vi "Working Window.vi"(8 "error in (no error)":errorcluster, 10 "file path":path=path "D:/Projects/Personal/Multi-LabVIEW-Selector/Multi-LabVIEW Selector.lvproj" caption="打开文件路径", 11 "DB Ref":refnum<class "SharedData.lvclass">) -> (0 "error out":errorcluster, 3 "DB Ref (dup)":refnum<class "SharedData.lvclass">)   [LabVIEW 2014]
uses:
  control/DEF-LabVIEW INFO.ctl
  <vilib>/NEVSTOP/Shared Data Library/SharedData/SharedData.lvclass
  control/DEF-State.ctl
  <vilib>/NEVSTOP/Shared Data Library/SharedData/SharedData.lvclass/SharedData.ctl
  <vilib>/NEVSTOP/Shared Data Library/SharedData/Data operation/_int32.vi
  <vilib>/NEVSTOP/Shared Data Library/SharedData/Data operation/_variant.vi
  <vilib>/NEVSTOP/Shared Data Library/SharedData/support/_[error50002]Invalid DataType.vi
  <vilib>/NEVSTOP/Shared Data Library/SharedData/support/_[error50001]Can't Found Value.vi
  <vilib>/NEVSTOP/Shared Data Library/SharedData/support/_[error50000]Invalid DB REF.vi
  <vilib>/Utility/error.llb/Trim Whitespace.vi
panel:
  out "Symbol Found?":bool
  out "Selected Version":string
  out "Version List":string[](array[string])
  out "Symbol Path":path
  out "Symbol Version":string
  out "LabVIEW Info":T1[](array[typedef])
  in  "Cancel":bool
  in  "OK":bool
  in  "LabVIEW List":string(combo)
  out "CMD line":string caption="命令行参数"
  # "主界面，所有的界面操作都产生消息，推送给Message Framework 处理。"
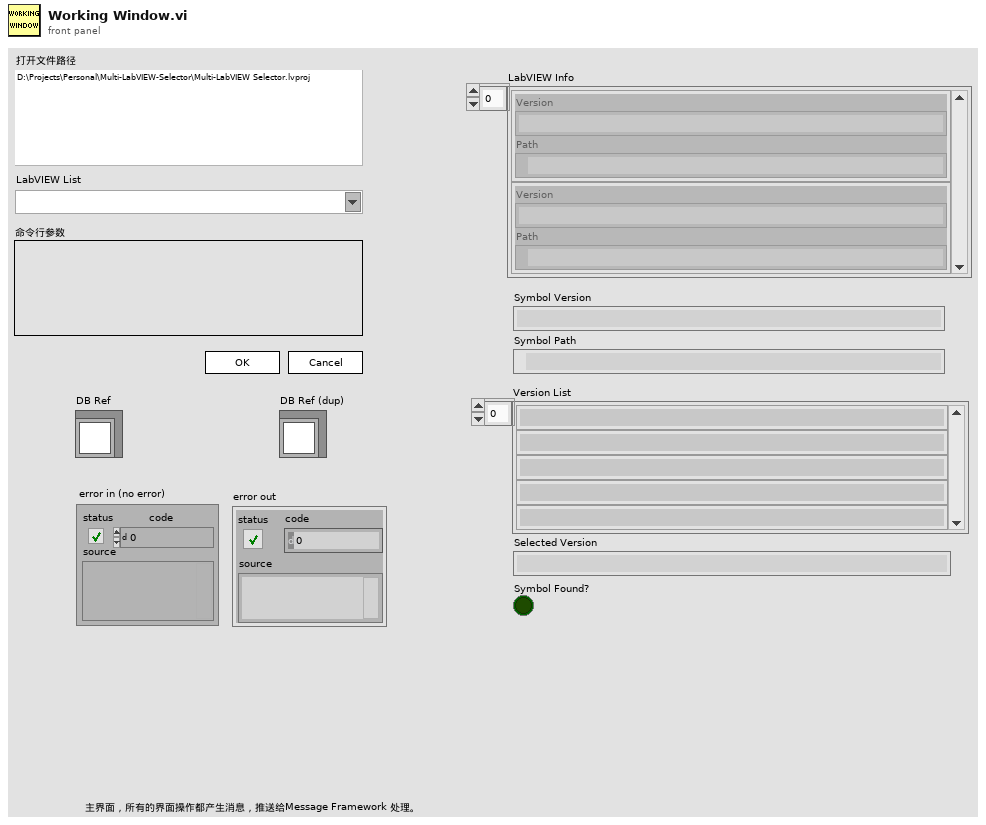
[diagram p1: front panel]
types:
  T1 = typedef "DEF-LabVIEW INFO.ctl" = cluster{"Version":string, "Path":path}
  T2 = typedef "DEF-State.ctl" = enum16{"Get Project Path", "Get Installed LabVIEW Version", "Find New Symbol", "Find Old Symbol", "Replace with New Symbol", "Check If The Symbol Version Exist", "Waiting for User Selection", "Display Information", "Get CMD", "Display CMD", "Excute CMD", "Exit"}
  T3 = cluster{"DB Ref":refnum<class "SharedData.lvclass">, "Project Path":path, "LabVIEW Info":T1[], "Symbol Version":string, "Symbol Path":path, "Version List":string[], "Selected Version":string, "Symbol Found?":bool, "CMD line":string}
  T4 = enum8{"Enabled", "Disabled", "Disabled and Grayed Out"}
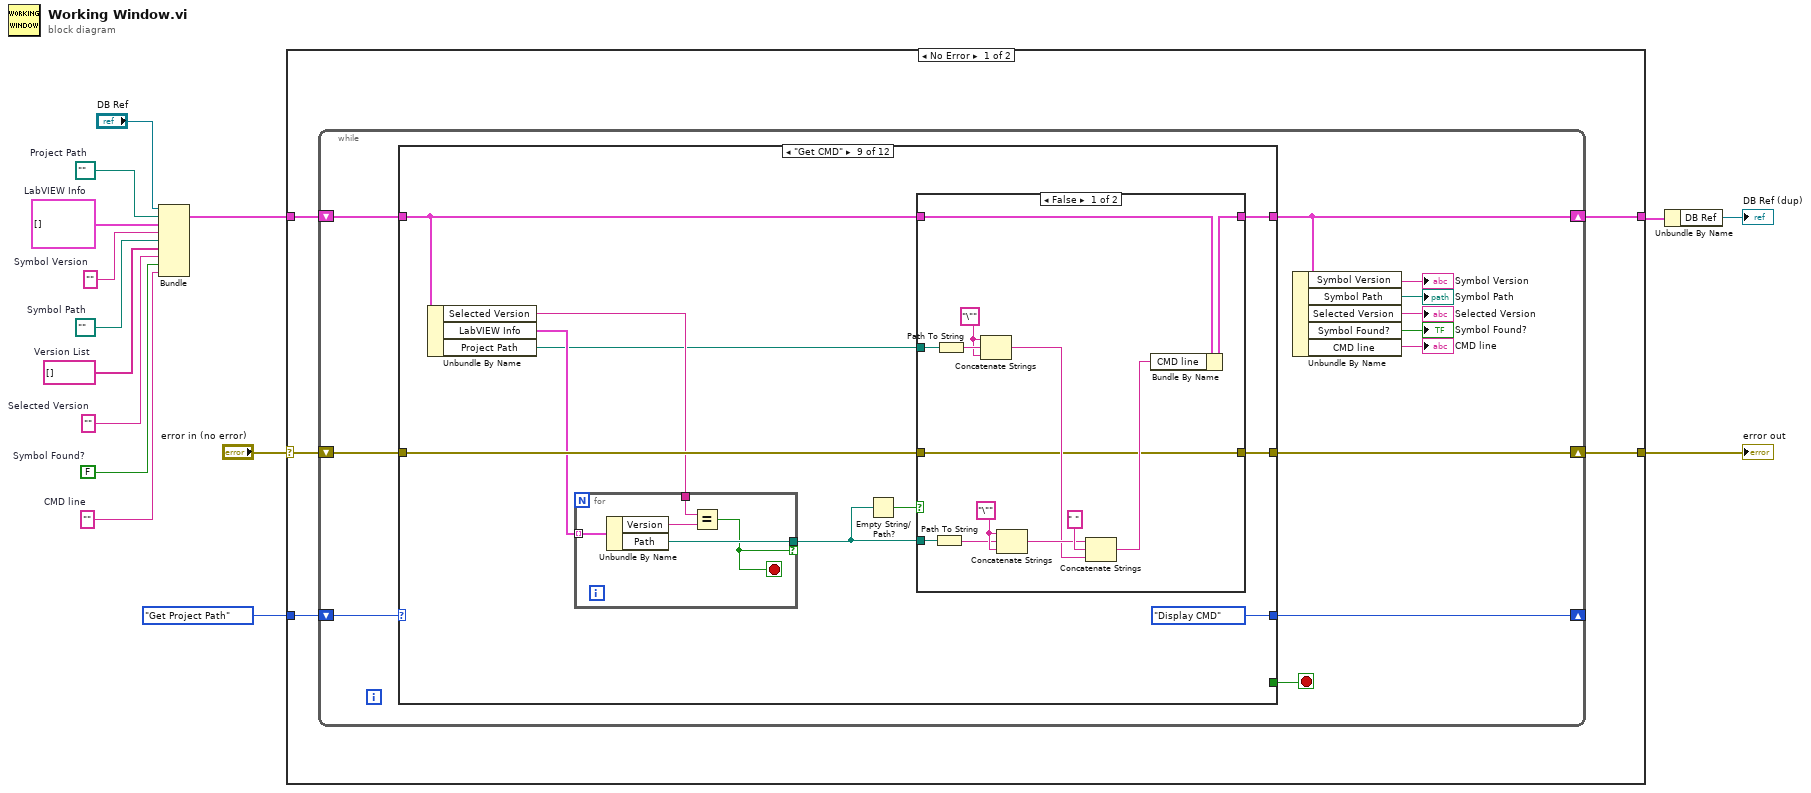
[diagram p0: block diagram]
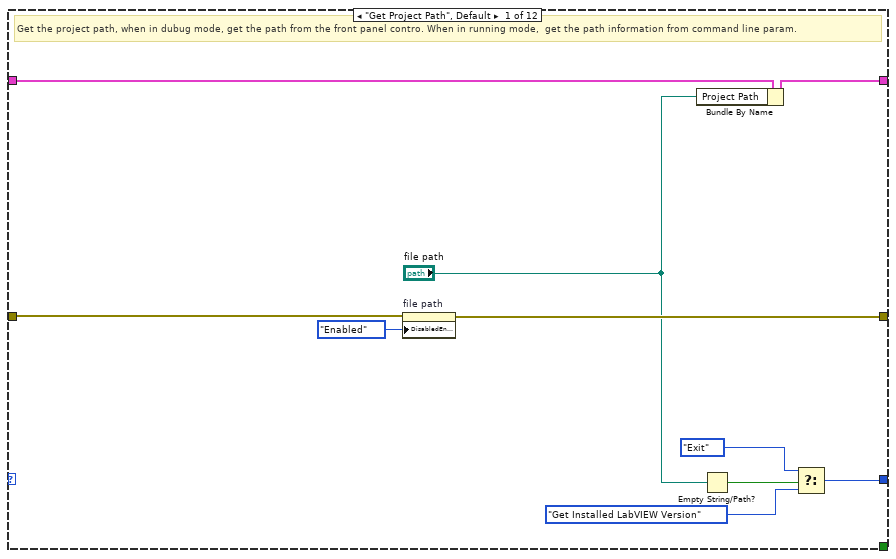
[diagram p2: hidden frame]
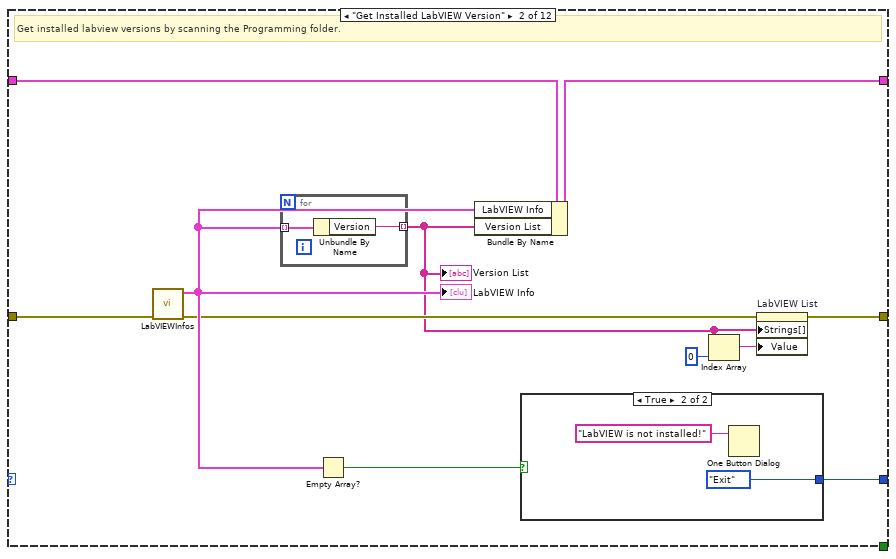
[diagram p3: hidden frame]
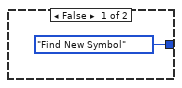
[diagram p4: hidden frame]
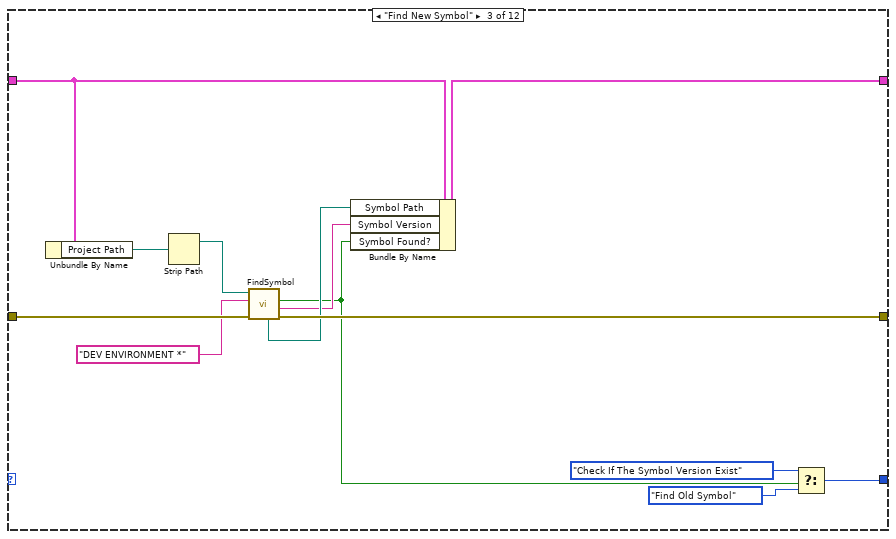
[diagram p5: hidden frame]
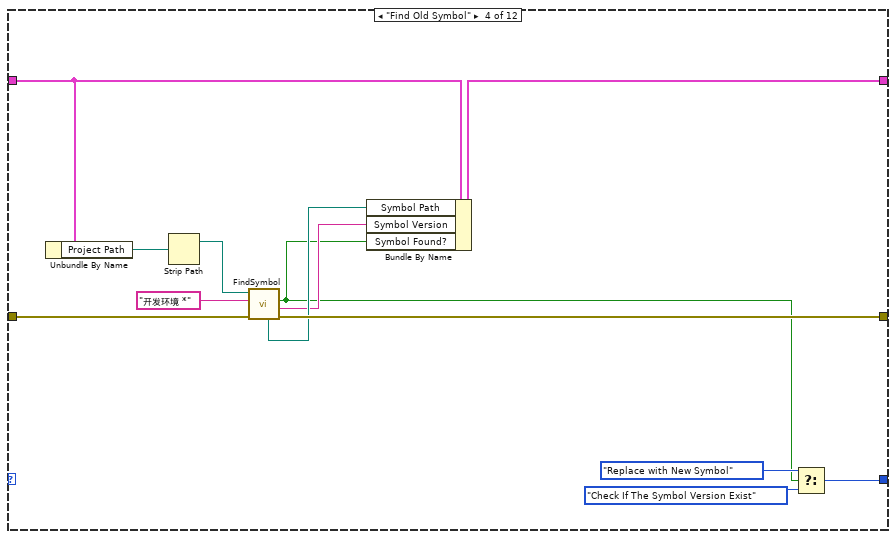
[diagram p6: hidden frame]
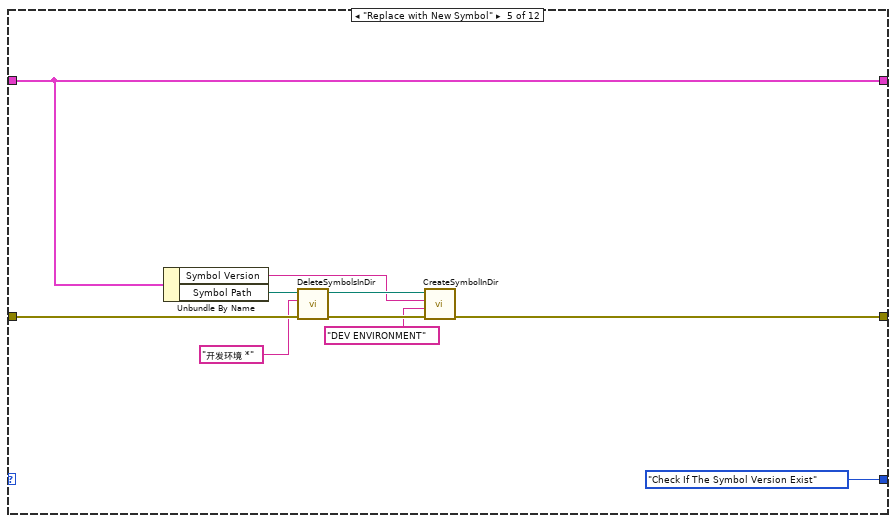
[diagram p7: hidden frame]
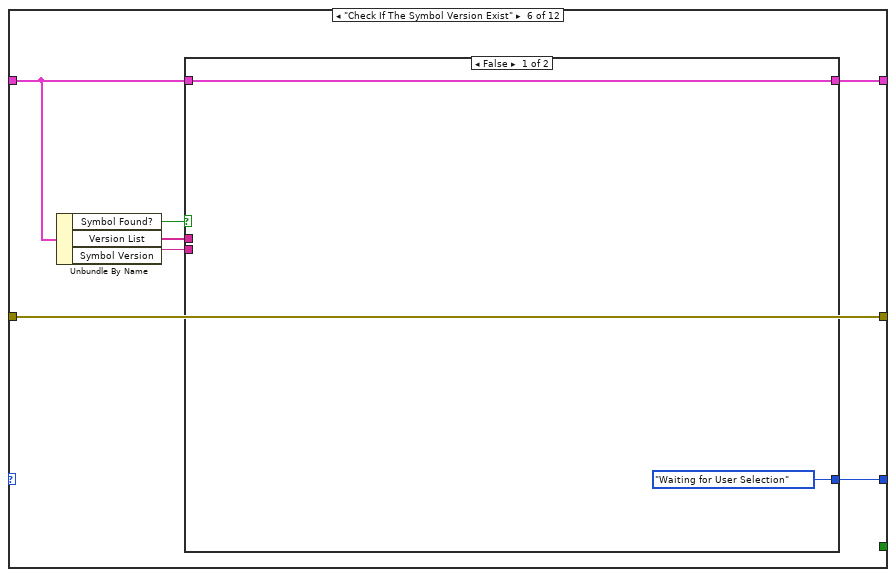
[diagram p8: hidden frame]
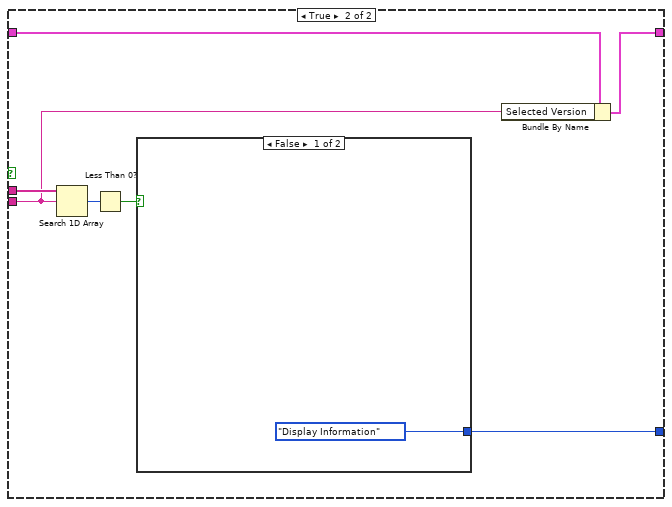
[diagram p9: hidden frame]
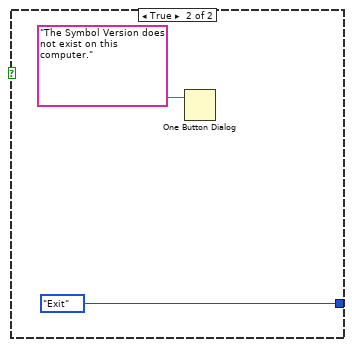
[diagram p10: hidden frame]
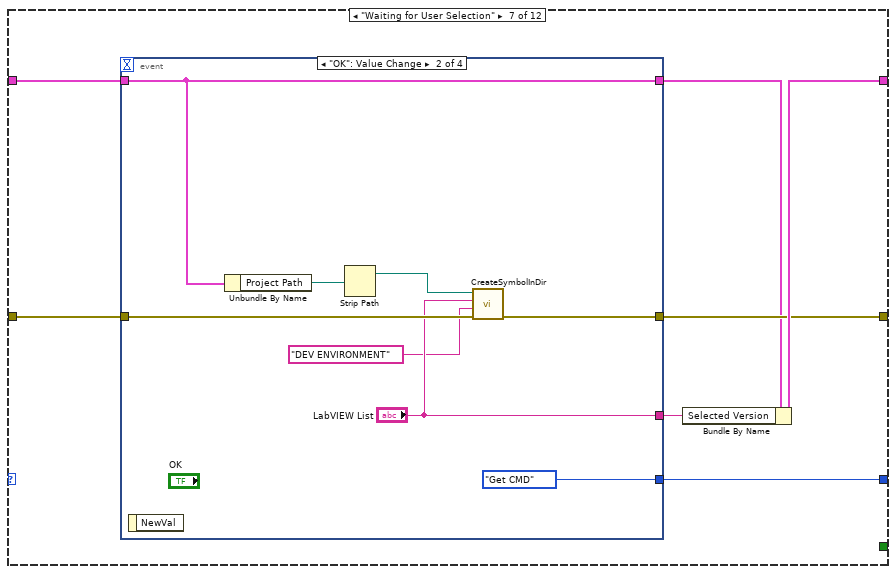
[diagram p11: hidden frame]
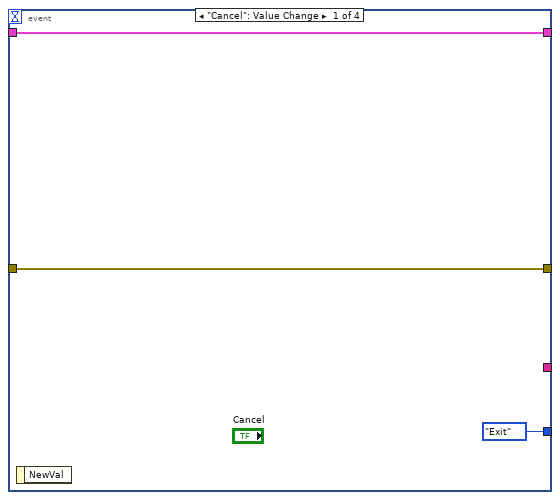
[diagram p12: hidden frame]
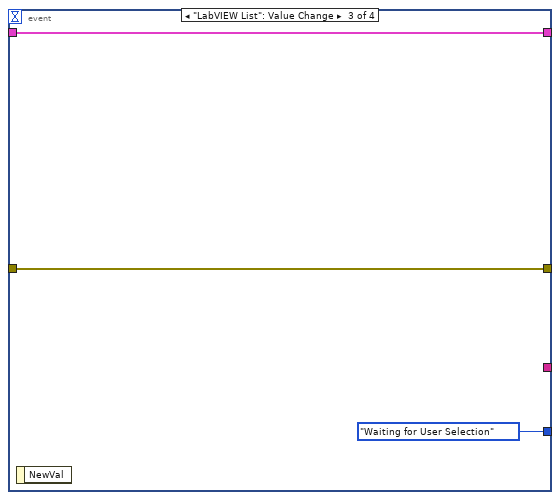
[diagram p13: hidden frame]
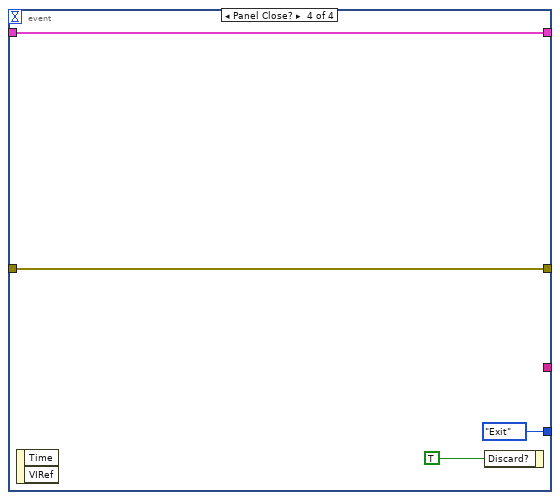
[diagram p14: hidden frame]
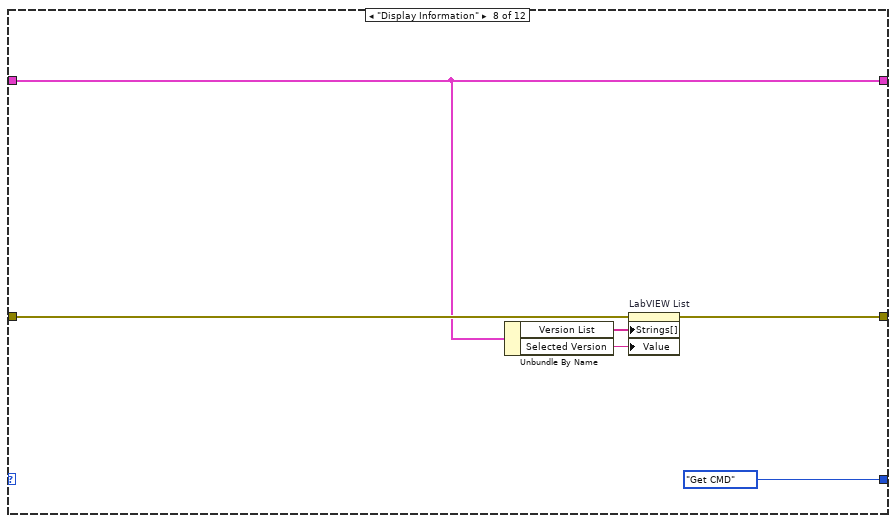
[diagram p15: hidden frame]
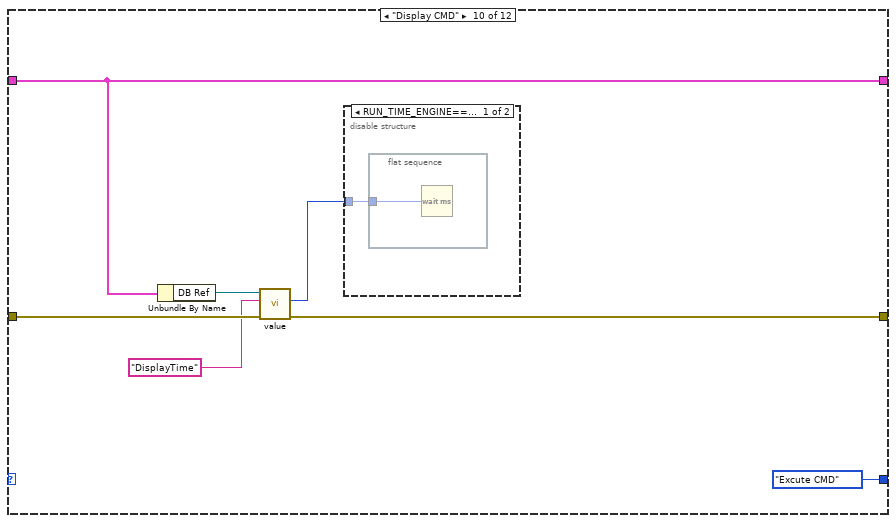
[diagram p17: hidden frame]
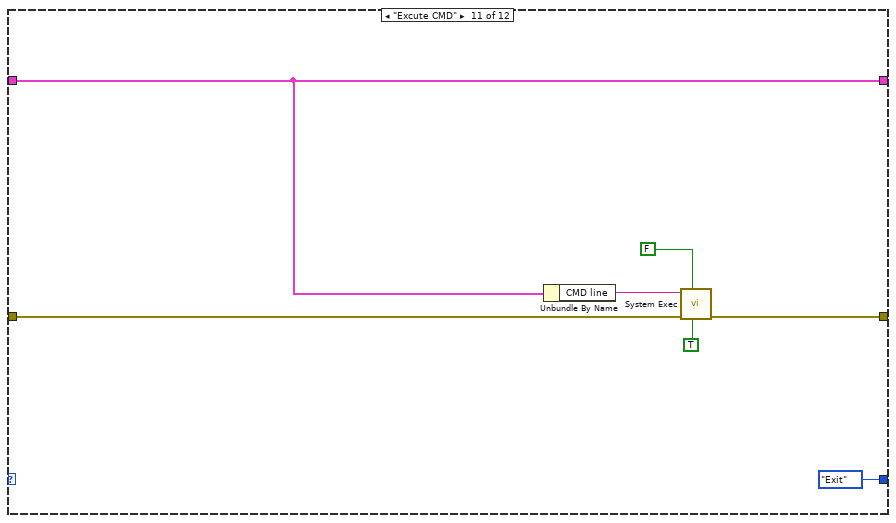
[diagram p19: hidden frame]
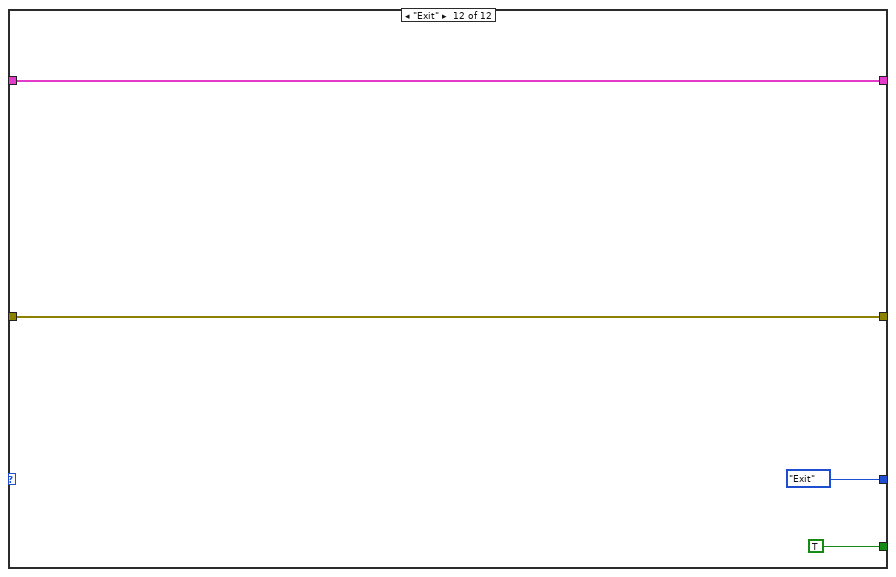
[diagram p20: hidden frame]
diagram:
  w7 = ""  # CMD line
  w8 = FALSE  # Symbol Found?
  w9 = ""  # Selected Version
  w10 = string[] []  # Version List
  w11 = path ""  # Symbol Path
  w12 = ""  # Symbol Version
  w13 = path ""  # Project Path
  w15 = T1[] []  # LabVIEW Info
  n1 = Bundle("DB Ref"="DB Ref", "Project Path"=w13, "LabVIEW Info"=w15, "Symbol Version"=w12, "Symbol Path"=w11, "Version List"=w10, "Selected Version"=w9, "Symbol Found?"=w8, "CMD line"=w7) -> (w14:T3)  [unwired: 1 in]
  n2 = case shown="No Error" "error in (no error)" {
    selector: "error in (no error)" -> [w19 w196]
    tunnel: w14 -> [w20 w195]
    tunnel: [w18 w196] -> w4
    tunnel: [w17 w195] -> w3
    tunnel: DEF-State."Get Project Path" -> [w16 _]
    frame No Error {
      n3 = while {
        shift-right: [w29] -> w18
        shift-left: w19 -> [w30]
        shift-right: [w28] -> _
        shift-left: w16 -> [w32]
        shift-right: [w26] -> w17
        shift-left: w20 -> [w27]
        stop <- w31 stop-if-true
        n4 = case shown="\"Get CMD\"" w32 {
          tunnel: [_ _ _ _ _ _ _ _ _ _ _ TRUE] -> w31
          tunnel: w30 -> [w41 w53 w69 w82 w94 w99 w117 w143 w154 w179 w187 w191]
          tunnel: [w42 w44 w65 w77 w89 w99 w116 w144 w153 w176 w188 w191] -> w29
          tunnel: [w39 w49 w66 w78 DEF-State."Check If The Symbol Version Exist" w98 w118 DEF-State."Get CMD" DEF-State."Display CMD" DEF-State."Excute CMD" DEF-State."Exit" DEF-State."Exit"] -> w28
          tunnel: w27 -> [w36 w52 w64 w76 w93 w96 w115 w142 w146 w180 w185 w192]
          tunnel: [w35 w51 w62 w74 w93 w95 w120 w142 w145 w180 w185 w192] -> w26
          frame "Get Project Path", Default {
            # "Get the project path, when in dubug mode, get the path from the front panel contro. When in running mode,  get the path information from command line param."
            n5 = property on="file path" class="Path"(error in=w41, "DisabledEnum"=T4."Enabled" ("Disabled")) -> (error out=w42:errorcluster)  [unwired: 1 in, 1 out]
            n6 = Bundle By Name(cluster=w36, "Project Path"="file path") -> (w35:T3)
            n7 = Empty String/Path?(string/path="file path") -> (empty?=w40:bool)
            n8 = Select(t=DEF-State."Exit", s=w40, f=DEF-State."Get Installed LabVIEW Version") -> (s? t:f=w39:T2)
          }
          frame "Get Installed LabVIEW Version" {
            # "Get installed labview versions by scanning the Programming folder."
            n9 = call "LabVIEWInfos.vi"("error in (no error)"=w53) -> ("error out"=w45:errorcluster, "LabVIEW Info"=w48:T1[])  [unwired: 9 in]
            "LabVIEW Info" <- w48
            n10 = for {
              tunnel: w48 -> [w55] mode=indexing
              tunnel: [w54] -> w43 mode=indexing
              n11 = Unbundle By Name(w55) -> ("Version"=w54:string)
            }
            "Version List" <- w43
            n12 = Empty Array?(array=w48) -> (empty?=w50:bool)
            n13 = Bundle By Name(cluster=w52, "LabVIEW Info"=w48, "Version List"=w43) -> (w51:T3)
            n14 = case shown="True" w50 {
              tunnel: [DEF-State."Find New Symbol" DEF-State."Exit"] -> w49
              frame False {
              }
              frame True {
                n15 = One Button Dialog(message="LabVIEW is not installed!") -> ()  [unwired: 1 in, 1 out]
              }
            }
            n16 = Index Array(array=w43, index=0) -> (element=w46:string)
            n17 = property on="LabVIEW List" class="CmbBox"(error in=w45, "Strings[]"=w43, "Value"=w46) -> (error out=w44:errorcluster)  [unwired: 1 in, 1 out]
          }
          frame "Find New Symbol" {
            n18 = Unbundle By Name(w64) -> ("Project Path"=w71:path)
            n19 = Strip Path(path=w71) -> (stripped path=w70:path)  [unwired: 1 out]
            n20 = call "FindSymbol.vi"("error in (no error)"=w69, "pattern"="DEV ENVIRONMENT *" ("prefix"), "path"=w70) -> ("error out"=w65:errorcluster, "Version"=w61:string, "Exits?"=w59:bool, "found path"=w63:path)  [unwired: 4 in, 1 out]
            n21 = Bundle By Name(cluster=w64, "Symbol Path"=w63, "Symbol Version"=w61, "Symbol Found?"=w59) -> (w62:T3)
            n22 = Select(t=DEF-State."Check If The Symbol Version Exist", s=w59, f=DEF-State."Find Old Symbol") -> (s? t:f=w66:T2)
          }
          frame "Find Old Symbol" {
            n23 = Unbundle By Name(w76) -> ("Project Path"=w84:path)
            n24 = Strip Path(path=w84) -> (stripped path=w83:path)  [unwired: 1 out]
            n25 = call "FindSymbol.vi"("error in (no error)"=w82, "pattern"="开发环境 *", "path"=w83) -> ("error out"=w77:errorcluster, "Version"=w73:string, "Exits?"=w72:bool, "found path"=w75:path)  [unwired: 4 in, 1 out]
            n26 = Bundle By Name(cluster=w76, "Symbol Path"=w75, "Symbol Version"=w73, "Symbol Found?"=w72) -> (w74:T3)
            n27 = Select(t=DEF-State."Replace with New Symbol", s=w72, f=DEF-State."Check If The Symbol Version Exist") -> (s? t:f=w78:T2)
          }
          frame "Replace with New Symbol" {
            n28 = Unbundle By Name(w93) -> ("Symbol Version"=w87:string, "Symbol Path"=w92:path)
            n29 = call "DeleteSymbolsInDir.vi"("error in (no error)"=w94, "pattern"="开发环境 *", "dup path"=w92) -> ("error in (no error) (dup)"=w90:errorcluster, "dup path (dup)"=w88:path)  [unwired: 7 in]
            n30 = call "CreateSymbolInDir.vi"("error in"=w90, "prefix"="DEV ENVIRONMENT", "Name"=w87, "Path"=w88) -> ("error out"=w89:errorcluster)  [unwired: 6 in, 1 out]
          }
          frame "Check If The Symbol Version Exist" {
            n31 = Unbundle By Name(w96) -> ("Symbol Found?"=w97:bool, "Version List"=w101:string[], "Symbol Version"=w100:string)
            n32 = case shown="False" w97 {
              tunnel: w101 -> [_ w109]
              tunnel: w100 -> [_ w104]
              tunnel: [DEF-State."Waiting for User Selection" w108] -> w98
              tunnel: w96 -> [w102 w106]
              tunnel: [w102 w105] -> w95
              frame False {
              }
              frame True {
                n33 = Search 1D Array(1D array=w109, element=w104) -> (index of element=w110:i32)  [unwired: 1 in]
                n34 = Less Than 0?(x=w110) -> (x < 0?=w107:bool)
                n35 = case shown="False" w107 {
                  tunnel: [DEF-State."Display Information" DEF-State."Exit"] -> w108
                  frame False {
                  }
                  frame True {
                    n36 = One Button Dialog(message="The Symbol Version does not exist on this computer.") -> ()  [unwired: 1 in, 1 out]
                  }
                }
                n37 = Bundle By Name(cluster=w106, "Selected Version"=w104) -> (w105:T3)
              }
            }
          }
          frame "Waiting for User Selection" {
            n38 = event shown="[1] \"OK\": Value Change" {
              selector: _ -> [_ _ _ _]
              dyn-events: _ -> [_ _ _ _]
              timeout: _ -> [_ _ _ _]
              tunnel: [_ "LabVIEW List" _ _] -> w119
              tunnel: [DEF-State."Exit" DEF-State."Get CMD" DEF-State."Waiting for User Selection" DEF-State."Exit"] -> w118
              tunnel: w117 -> [w122 w130 w133 w136]
              tunnel: [w122 w129 w133 w136] -> w116
              tunnel: w115 -> [w121 w128 w132 w135]
              tunnel: [w121 w128 w132 w135] -> w114
              event "Cancel": Value Change {
                n39 = event-data() -> ()  [unwired: 1 in, 1 out]
              }
              event "OK": Value Change {
                n40 = event-data() -> ()  [unwired: 1 in, 1 out]
                n41 = Unbundle By Name(w128) -> ("Project Path"=w127:path)
                n42 = Strip Path(path=w127) -> (stripped path=w126:path)  [unwired: 1 out]
                n43 = call "CreateSymbolInDir.vi"("error in"=w130, "prefix"="DEV ENVIRONMENT", "Name"="LabVIEW List", "Path"=w126) -> ("error out"=w129:errorcluster)  [unwired: 6 in, 1 out]
              }
              event "LabVIEW List": Value Change {
                n44 = event-data() -> ()  [unwired: 1 in, 1 out]
              }
              event Panel Close? {
                n45 = event-data() -> ()  [unwired: 1 in, 2 out]
                n46 = event-data("Discard?"=TRUE) -> ()  [unwired: 1 in, 1 out]
              }
            }
            n47 = Bundle By Name(cluster=w114, "Selected Version"=w119) -> (w120:T3)
          }
          frame "Display Information" {
            n48 = Unbundle By Name(w142) -> ("Version List"=w141:string[], "Selected Version"=w140:string)
            n49 = property on="LabVIEW List" class="CmbBox"(error in=w143, "Strings[]"=w141, "Value"=w140) -> (error out=w144:errorcluster)  [unwired: 1 in, 1 out]
          }
          frame "Get CMD" {
            n50 = Unbundle By Name(w146) -> ("Selected Version"=w150:string, "LabVIEW Info"=w149:T1[], "Project Path"=w147:path)
            n51 = for {
              tunnel: w149 -> [w174] mode=indexing
              tunnel: [w172] -> w152 if=w170
              tunnel: w150 -> [w171]
              stop <- w170 stop-if-true
              n52 = Unbundle By Name(w174) -> ("Version"=w173:string, "Path"=w172:path)
              n53 = Equal?(x=w171, y=w173) -> (x = y?=w170:bool)
            }
            n54 = Empty String/Path?(string/path=w152) -> (empty?=w151:bool)
            n55 = case shown="False" w151 {
              tunnel: w154 -> [w155 w169]
              tunnel: w152 -> [w167 _]
              tunnel: [w155 w169] -> w153
              tunnel: w147 -> [w159 _]
              tunnel: w146 -> [w158 w168]
              tunnel: [w157 w168] -> w145
              frame False {
                w164 = "\"" ("string")
                w165 = "\"" ("string")
                n56 = Path To String(path=w167) -> (string=w163:string)
                n57 = Path To String(path=w159) -> (string=w166:string)
                n58 = Concatenate Strings(w165, w166, w165) -> (w160:string)
                n59 = Concatenate Strings(w164, w163, w164) -> (w161:string)
                n60 = Concatenate Strings(w161, " " ("string"), w160) -> (w156:string)
                n61 = Bundle By Name(cluster=w158, "CMD line"=w156) -> (w157:T3)
              }
              frame True {
              }
            }
          }
          frame "Display CMD" {
            n62 = Unbundle By Name(w180) -> ("DB Ref"=w178:refnum<class "SharedData.lvclass">)
            n63 = call-poly <vilib>:"value.vi"("error in (no error)"=w179, "name"="DisplayTime", "DB Ref"=w178) -> ("error in (no error) (dup)"=w176:errorcluster, "value"=w177:i32)  [unwired: 6 in, 1 out]
            n64 = disable-structure shown="RUN_TIME_ENGINE==True" {
              disable-tunnel: w177 -> [w182 _]
              frame condition #0 {
                n65 = flat-sequence {
                  tunnel: w182 -> [w183]
                  frame #0 {
                    n66 = Wait (ms)(milliseconds to wait=w183) -> ()  [unwired: 1 out]
                  }
                }
              }
              frame condition #1 (active) {
              }
            }
          }
          frame "Excute CMD" {
            n67 = Unbundle By Name(w185) -> ("CMD line"=w184:string)
            n68 = call <vilib>:"System Exec.vi"("run minimized? (F)"=TRUE, "wait until completion? (T)"=FALSE, "error in (no error)"=w187, "command line"=w184) -> ("error out"=w188:errorcluster)  [unwired: 4 in, 3 out]
          }
          frame "Exit" {
          }
        }
        n69 = Unbundle By Name(w26) -> ("Symbol Version"=→"Symbol Version":string, "Symbol Path"=→"Symbol Path":path, "Selected Version"=→"Selected Version":string, "Symbol Found?"=→"Symbol Found?":bool, "CMD line"=→"CMD line":string)
      }
    }
    frame Error {
    }
  }
  "error out" <- w4
  n70 = Unbundle By Name(w3) -> ("DB Ref"=→"DB Ref (dup)":refnum<class "SharedData.lvclass">)
